vi "Create TCP Master.vi"(8 "error in":errorcluster, 9 "connect timeout ms":i32=10000, 10 "port (502)":u16=502, 11 "address":string) -> (0 "error out":errorcluster, 3 "TCP master instance":refnum<class "Modbus Master.lvclass">)   [LabVIEW 2012, in "API Main.lvlib"]
doc: "Creates a standard TCP master using an IP transmission data unit. This instance looks for a slave at the <B>address</B> and <B>port</B> specified."
uses:
  API Main.lvlib
  Master/Modbus Master.lvclass
  Transmission Data Unit/IP/IP Data Unit.lvclass
  Master Function Definition/Master Function Definition.lvclass
  Network Protocol/Network Master/TCP/TCP Master.lvclass
  Network Protocol/Network Master/TCP/TCP Master.lvclass/TCP Master.ctl
  Transmission Data Unit/Transmission Data Unit.lvclass/Transmission Data Unit.ctl
  Modbus API.lvclass/Modbus API.ctl
  Master/Modbus Master.lvclass/Modbus Master.ctl
  Network Protocol/Network Master/TCP/Write Address.vi
  Network Protocol/Network Master/TCP/Write Port.vi
  Network Protocol/Network Master/TCP/Write connect timeout ms.vi
  Modbus API.lvclass
  Transmission Data Unit/Transmission Data Unit.lvclass
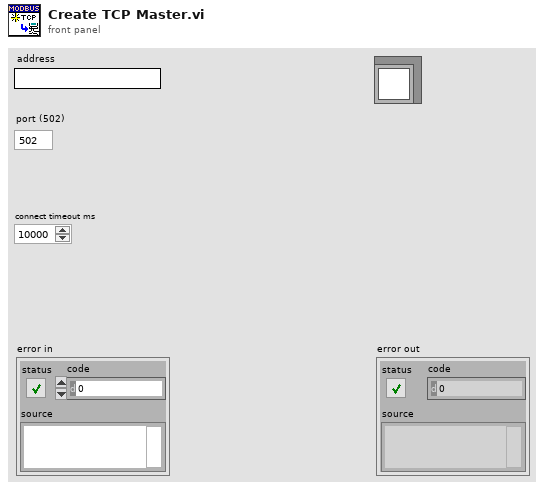
[diagram p1: front panel]
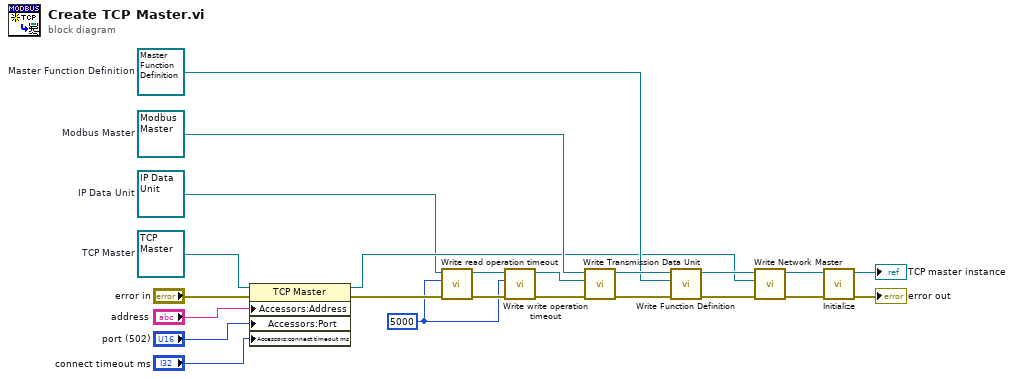
[diagram p0: block diagram]
diagram:
  w2 = 5000 ("read operation timeout")
  w23 = refnum<class "TCP Master.lvclass"> refnum  # TCP Master
  w14 = refnum<class "Master Function Definition.lvclass"> refnum  # Master Function Definition
  w4 = refnum<class "IP Data Unit.lvclass"> refnum  # IP Data Unit
  w17 = refnum<class "Modbus Master.lvclass"> refnum  # Modbus Master
  n1 = property class="TCP Master"(reference=w23, error in="error in", "Accessors:Address"="address", "Accessors:Port"="port (502)", "Accessors:connect timeout ms"="connect timeout ms") -> (reference out=w11:refnum<class "TCP Master.lvclass">, error out=w3:errorcluster)
  n2 = call "Write read operation timeout.vi"("error in (no error)"=w3, "read operation timeout"=w2, "transmission data unit in"=w4) -> ("error out"=w7:errorcluster, "transmission data unit out"=w8:refnum<class "IP Data Unit.lvclass">)  [unwired: 7 in]
  n3 = call "Write write operation timeout.vi"("error in (no error)"=w7, "write operation timeout"=w2, "transmission data unit in"=w8) -> ("error out"=w6:errorcluster, "transmission data unit out"=w5:refnum<class "IP Data Unit.lvclass">)  [unwired: 7 in]
  n4 = call "Write Transmission Data Unit.vi"("error in"=w6, "transmission data unit"=w5, "Modbus instance in"=w17) -> ("error out"=w15:errorcluster, "Modbus instance out"=w16:refnum<class "Modbus Master.lvclass">)  [unwired: 7 in]
  n5 = call "Write Function Definition.vi"("error in"=w15, "master function definition"=w14, "Modbus master in"=w16) -> ("error out"=w12:errorcluster, "Modbus master out"=w13:refnum<class "Modbus Master.lvclass">)  [unwired: 7 in]
  n6 = call "Write Network Master.vi"("error in"=w12, "network master"=w11, "Modbus master in"=w13) -> ("error out"=w10:errorcluster, "Modbus master out"=w9:refnum<class "Modbus Master.lvclass">)  [unwired: 7 in]
  n7 = call-dynamic "Initialize.vi"("error in"=w10, "Modbus master in"=w9) -> ("error out"=→"error out":errorcluster, "Modbus master out"=→"TCP master instance":refnum<class "Modbus Master.lvclass">)  [unwired: 8 in]
